vi "Set Endpoint Configuration.vi"(8 "error in":errorcluster, 9 "configuration":T1, 10 "endpoint":string, 11 "endpoint configuration in":T2 format="%.0x") -> (0 "error out":errorcluster, 3 "endpoint configuration out":T2 format="%.0x")   [LabVIEW 2020, in "SLSC Switch Scripting.lvlib"]
doc: "Sets the configuration for one endpoint. The configuration restricts how the endpoint can be used, including reserving it for internal routing (configuration) and preventing it from being connected to other endpoints (source)."
uses:
  SLSC Switch Scripting.lvlib
  <vilib>/NI VeriStand/Custom Device API/Custom Device Item Ref.ctl
  Shared/Endpoint Configuration Enum.ctl
  <vilib>/NI VeriStand/Custom Device API/Custom Device API.lvlib
  Dependencies.llb/SLSC Switch Shared.lvlib
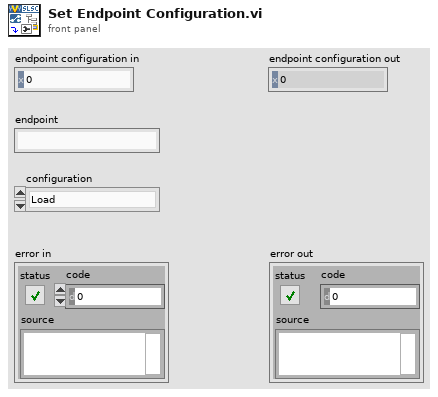
[diagram p1: front panel]
types:
  T1 = typedef "SLSC Switch Shared.lvlib/Endpoint Configuration Enum.ctl" = enum16{"Load", "Source", "Configuration"}
  T2 = typedef "Custom Device API.lvlib/Custom Device Item Ref.ctl" = u64
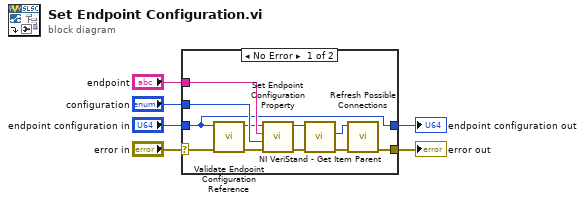
[diagram p0: block diagram]
diagram:
  n1 = case shown="No Error" "error in" {
    selector: "error in" -> [w16 w19]
    tunnel: "endpoint" -> [w17 _]
    tunnel: "configuration" -> [w15 _]
    tunnel: "endpoint configuration in" -> [w7 w18]
    tunnel: [w8 w19] -> w2
    tunnel: [w7 w18] -> w1
    frame No Error {
      n2 = call "Validate Endpoint Configuration Reference.vi"("error in"=w16, "endpoint configuration in"=w7) -> ("error out"=w14:errorcluster, "endpoint configuration out"=w13:T2)  [unwired: 8 in]
      n3 = call "Set Endpoint Configuration Property.vi"("error in"=w14, "configuration"=w15, "endpoint"=w17, "endpoint configuration in"=w13) -> ("error out"=w9:errorcluster, "endpoint configuration out"=w10:T2)  [unwired: 6 in]
      n4 = call <vilib>:"NI VeriStand - Get Item Parent.vi"("error in (no error)"=w9, "Item Ref in"=w10) -> ("error out"=w11:errorcluster, "Parent Ref"=w12:T2)  [unwired: 6 in, 2 out]
      n5 = call "Refresh Possible Connections.vi"("error in"=w11, "slsc switch custom device in"=w12) -> ("error out"=w8:errorcluster)  [unwired: 8 in, 1 out]
    }
    frame Error {
    }
  }
  "error out" <- w2
  "endpoint configuration out" <- w1
